vi "小时数组插时间戳和空值.vi"(0 "多参数":string[][](array[string]), 1 "待插值":string[][](array[string])) -> (8 "新输出":string[][](array[string]))   [LabVIEW 2016]
panel:
  out "数值 3":i32
  out "元素索引":i32
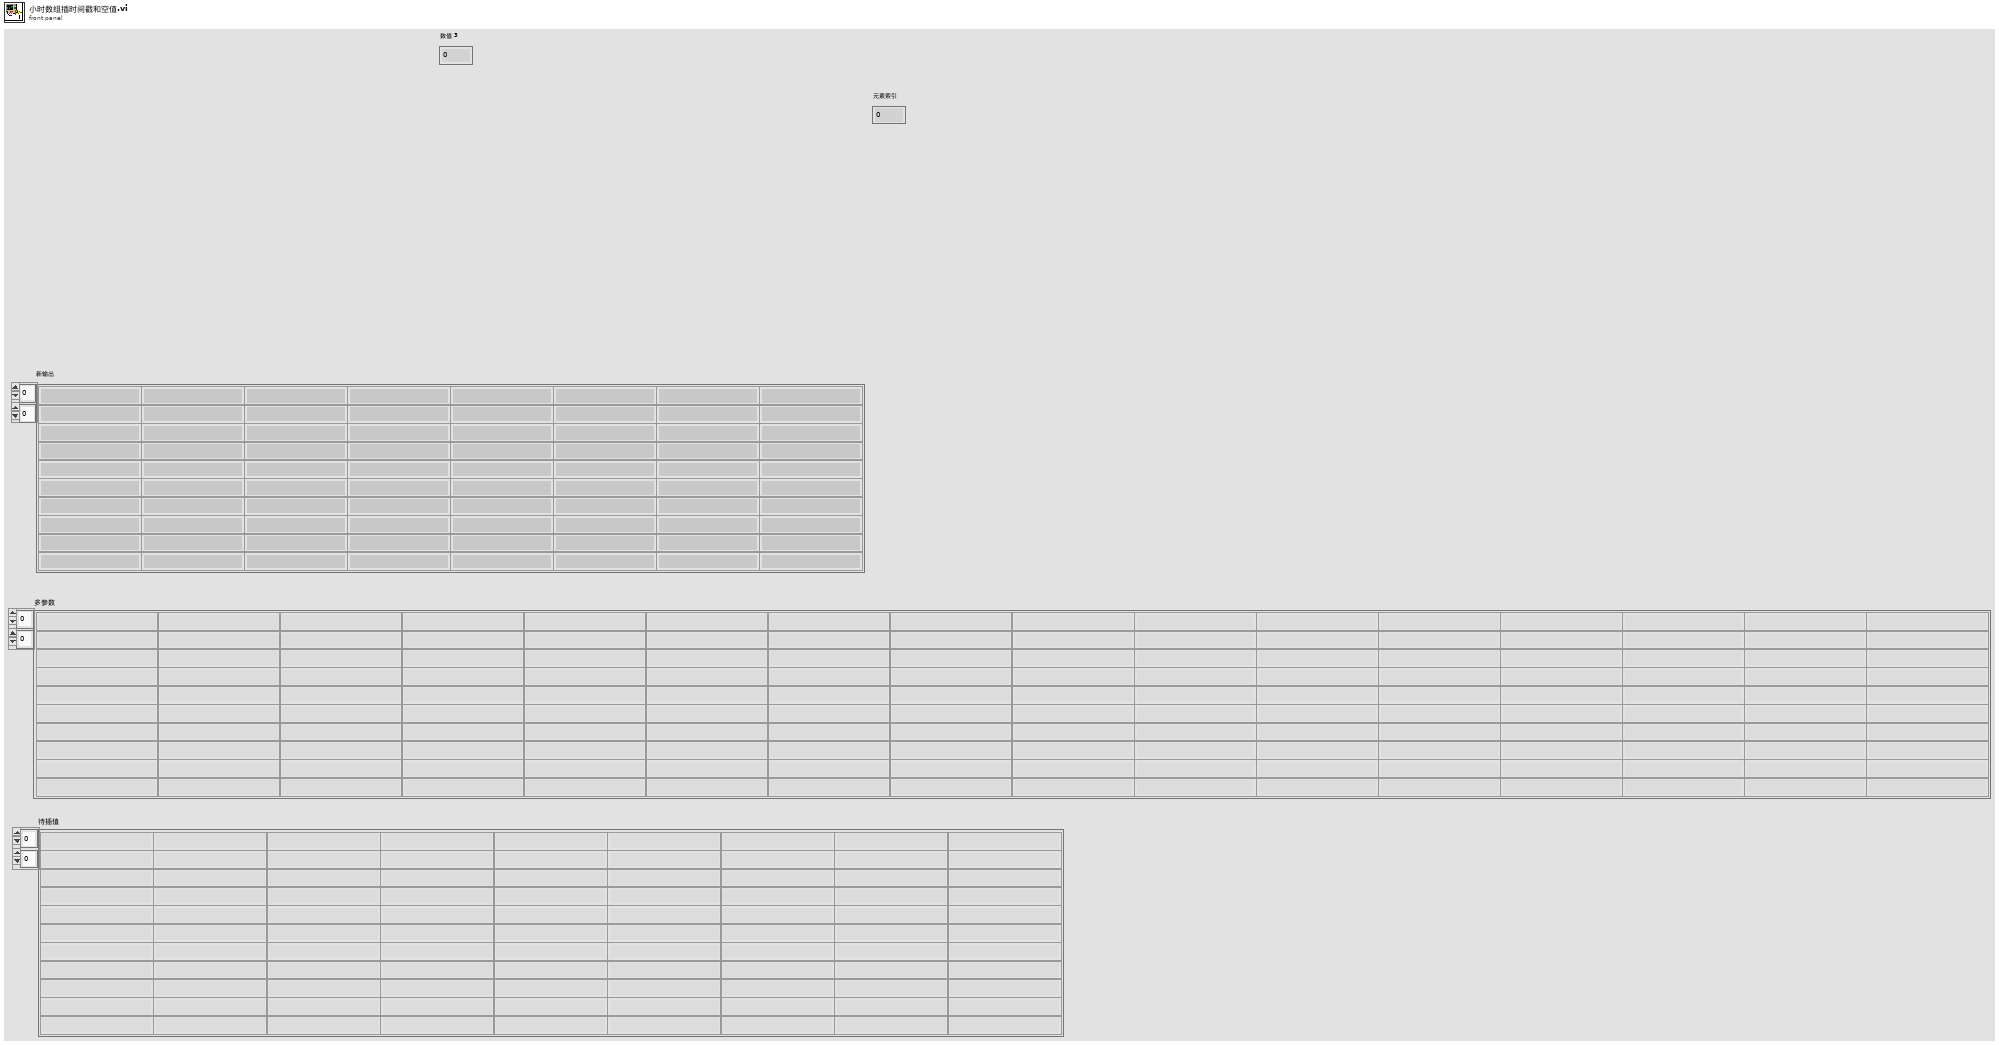
[diagram p1: front panel]
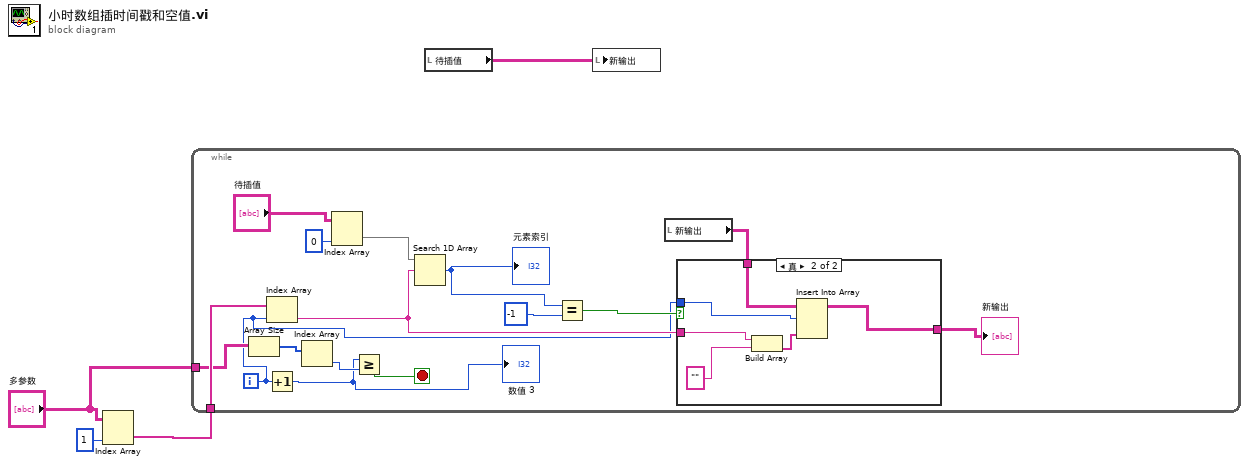
[diagram p0: block diagram]
diagram:
  n1 = Index Array(array="多参数", index (col)=1 ("禁用的索引 (列)")) -> (element=w3:string[])  [unwired: 1 in]
  n2 = while {
    tunnel: w3 -> [w14]
    tunnel: "多参数" -> [w12]
    i -> [w6]
    stop <- w10 stop-if-true
    n3 = Array Size(array=w12) -> (size(s)=w11:i32[])
    n4 = Index Array(array=w14, index=w6) -> (element=w15:string)
    n5 = Increment(x=w6) -> (x+1=w7:i32)
    "数值 3" <- w7
    n6 = Index Array(array=w11) -> (element=w8:i32)  [unwired: 1 in]
    n7 = Index Array(array="待插值", index (col)=0 ("禁用的索引 (列)")) -> (element=w13:string[])  [unwired: 1 in]
    n8 = Greater Or Equal?(x=w7, y=w8) -> (x >= y?=w10:bool)
    n9 = Search 1D Array(1D array=w13, element=w15) -> (index of element=w19:i32)  [unwired: 1 in]
    "元素索引" <- w19
    n10 = Equal?(x=w19, y=-1) -> (x = y?=w17:bool)
    n11 = local read "新输出"() -> (w5:string[][])
    n12 = case shown="真" w17 {
      tunnel: w5 -> [w21 w27]
      tunnel: w15 -> [_ w22]
      tunnel: w6 -> [_ w25]
      tunnel: [w21 w24] -> w9
      frame False {
      }
      frame True {
        n13 = Build Array(w22, "" ("元素")) -> (w26:string[])
        n14 = Insert Into Array(array=w27, index (row)=w25, new element=w26) -> (w24:string[][])  [unwired: 1 in]
      }
    }
    "新输出" <- w9
  }
  n15 = local read "待插值"() -> (w1:string[][])
  n16 = local write "新输出"(w1) -> ()
